vi "FloatPanel.vi"(8 "error in (no error)":errorcluster caption="错误输入（无错误）", 11 "PanelDataNode 输入":refnum<class "PanelDataNode.lvclass"> caption="DNL_LabVIEW Object in") -> (0 "error out":errorcluster caption="错误输出", 3 "PanelDataNode 输出":refnum<class "PanelDataNode.lvclass"> caption="DNL_LabVIEW Object out")   [LabVIEW 2016, in "PanelDataNode.lvclass"]
uses:
  PanelDataNode.lvclass
  PanelDataNode.lvclass/PanelDataNode.ctl
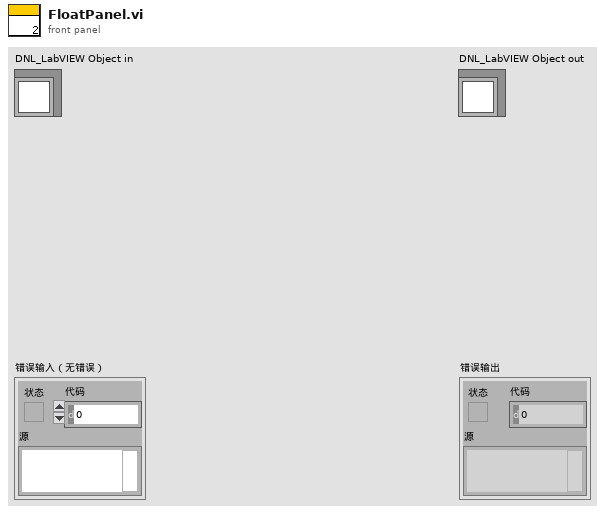
[diagram p1: front panel]
types:
  T1 = enum32{"Invalid", "Standard", "Closed", "Hidden", "Minimized", "Maximized"}
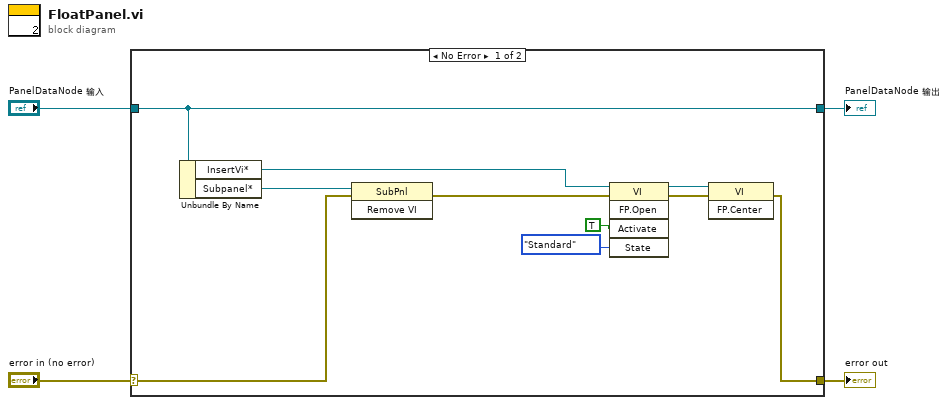
[diagram p0: block diagram]
diagram:
  n1 = case shown="No Error" "error in (no error)" {
    selector: "error in (no error)" -> [w12 w16]
    tunnel: [w5 w16] -> w3
    tunnel: [w14 w15] -> w1
    tunnel: "PanelDataNode 输入" -> [w14 w15]
    frame No Error {
      n2 = Unbundle By Name(w14) -> ("InsertVi*"=w11:refnum<vi>, "Subpanel*"=w13:refnum<vi>)
      n3 = invoke class="SubPnl" method="Remove VI"(reference=w13, error in=w12) -> (error out=w10:errorcluster)  [unwired: 1 in, 2 out]
      n4 = invoke class="VI" method="FP.Open"(reference=w11, error in=w10, "Activate"=TRUE ("激活？"), "State"=T1."Standard" ("州")) -> (reference out=w7:refnum<vi>, error out=w6:errorcluster)  [unwired: 1 in, 3 out]
      n5 = invoke class="VI" method="FP.Center"(reference=w7, error in=w6) -> (error out=w5:errorcluster)  [unwired: 1 in, 2 out]
    }
    frame Error {
    }
  }
  "error out" <- w3
  "PanelDataNode 输出" <- w1
